vi "Read String.vi"(8 "error in (no error)":errorcluster, 11 "String Message in":refnum<class "String Message.lvclass">) -> (0 "error out":errorcluster, 2 "String":string, 3 "String Message out":refnum<class "String Message.lvclass">)   [LabVIEW 2015, in "RDS Child Messages.lvlib" / "String Message.lvclass"]
uses:
  String Message.lvclass
  String Message.lvclass/String Message.ctl
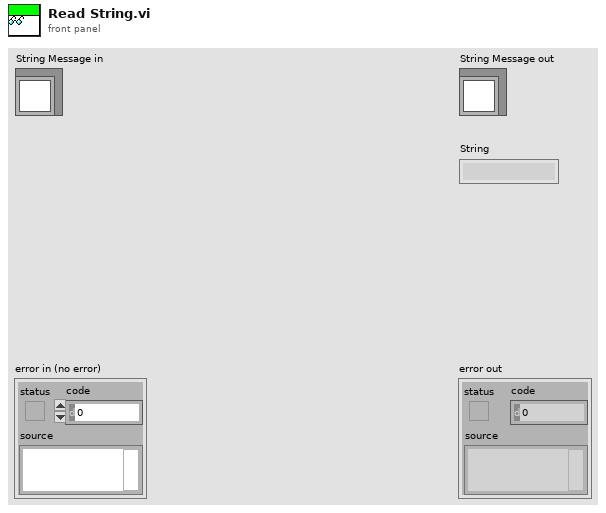
[diagram p1: front panel]
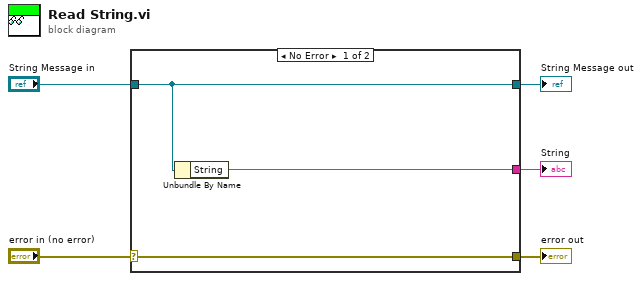
[diagram p0: block diagram]
diagram:
  n1 = case shown="No Error" "error in (no error)" {
    selector: "error in (no error)" -> [w8 w9]
    tunnel: [w8 w9] -> w4
    tunnel: [w7 w10] -> w2
    tunnel: "String Message in" -> [w7 w10]
    tunnel: [w6 _] -> w1
    frame No Error {
      n2 = Unbundle By Name(w7) -> ("String"=w6:string)
    }
    frame Error {
    }
  }
  "error out" <- w4
  "String Message out" <- w2
  "String" <- w1
